vi "Initialization.vi"(8 "error in (no error)":errorcluster, 11 "RTL-SDR in":refnum<class "RTL-SDR.lvclass">) -> (0 "error out":errorcluster, 2 "rtlsdr Path":path, 3 "RTL-SDR out":refnum<class "RTL-SDR.lvclass">)   [LabVIEW 2015, in "RTL-SDR.lvclass"]
doc: "Created IvanLis by LabVIEW Portal\nProfile: http://labviewportal.org/memberlist.php?mode=viewprofile&u=987\neMail: IvanLisanov@gMail.com\nTelegram: https://t.me/IvanLis"
uses:
  RTL-SDR.lvclass
  RTL-SDR.lvclass/RTL-SDR.ctl
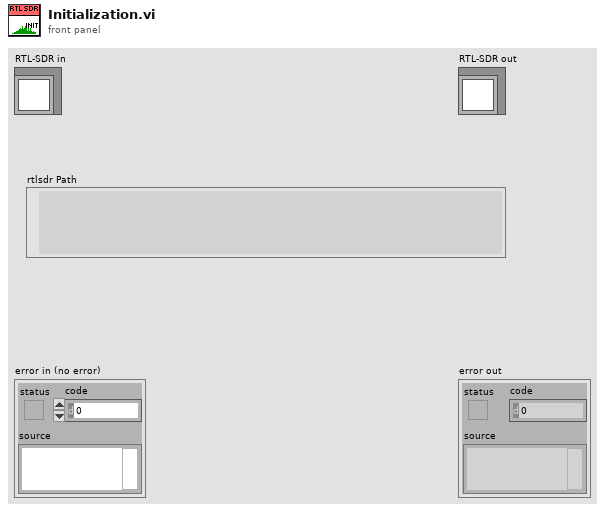
[diagram p1: front panel]
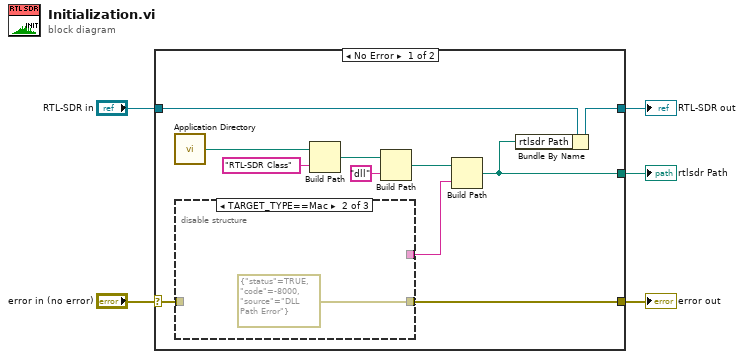
[diagram p0: block diagram]
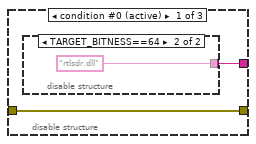
[diagram p2: hidden frame]
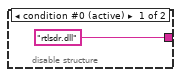
[diagram p3: hidden frame]
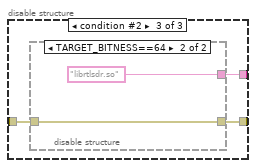
[diagram p4: hidden frame]
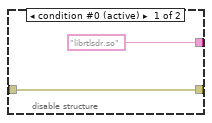
[diagram p5: hidden frame]
diagram:
  n1 = case shown="No Error" "error in (no error)" {
    selector: "error in (no error)" -> [w8 w30]
    tunnel: [w7 w30] -> w4
    tunnel: [w11 w29] -> w2
    tunnel: "RTL-SDR in" -> [w16 w29]
    tunnel: [w10 _] -> w1
    frame No Error {
      n2 = call <vilib>:"Application Directory.vi"() -> ("Application Directory"=w9:path)
      n3 = disable-structure shown="TARGET_TYPE==Mac" {
        disable-tunnel: w8 -> [w18 _ w24]
        disable-tunnel: [w18 errorcluster {"status"=TRUE, "code"=-8000, "source"="DLL Path Error"} ("error IO") w23] -> w7
        disable-tunnel: [w17 _ w22] -> w6
        frame condition #0 (active) {
          n4 = disable-structure shown="TARGET_BITNESS==64" {
            disable-tunnel: ["rtlsdr.dll" ("name or relative path") "rtlsdr.dll" ("name or relative path")] -> w17
            frame condition #0 (active) {
            }
            frame condition #1 {
            }
          }
        }
        frame condition #1 {
        }
        frame condition #2 {
          n5 = disable-structure shown="TARGET_BITNESS==64" {
            disable-tunnel: ["librtlsdr.so" ("name or relative path") "librtlsdr.so" ("name or relative path")] -> w22
            disable-tunnel: w24 -> [w25 w28]
            disable-tunnel: [w25 w28] -> w23
            frame condition #0 (active) {
            }
            frame condition #1 {
            }
          }
        }
      }
      n6 = Build Path(base path=w9, name or relative path="RTL-SDR Class") -> (appended path=w15:path)
      n7 = Build Path(base path=w15, name or relative path="dll") -> (appended path=w13:path)
      n8 = Build Path(base path=w13, name or relative path=w6) -> (appended path=w10:path)
      n9 = Bundle By Name(cluster=w16, "rtlsdr Path"=w10) -> (w11:refnum<class "RTL-SDR.lvclass">)
    }
    frame Error {
    }
  }
  "error out" <- w4
  "RTL-SDR out" <- w2
  "rtlsdr Path" <- w1
